vi "MB Param redefine.vi"(6 "conninfo":T1={"host"="localhost", "port"="5432", "client_encoding"="WIN1251", "dbname"="data", "user"="postgres", "password"=""}, 8 "error in (no error)":errorcluster, 9 "KFMTable":string="kfm_3", 10 "KFM param":string[](array[string]), 11 "MBs":refnum<class "Modbus Master CR.lvclass">[](array[class])) -> (0 "error":errorcluster, 3 "MBs out":refnum<class "Modbus Master CR.lvclass">[](array[class]))   [LabVIEW 2021]
uses:
  PostgreSQL/PostgreSQL2LabVIEW/ctl/Coninfo.ctl
  MB/Modbus Master CR.lvclass
  MBTCP Param/Typedefs/KFMParamColumns.ctl
  MBTCP Param/MBTCP Param.lvclass
  D:/my_projects/projects/Algorithms/Labview/21/Modbus_v2/MB Param/MB Param/MB Param.lvclass
  MB/Modbus Master CR.lvclass/Modbus Master CR.ctl
  MB Param.lvclass/MB Param.ctl
  MBTCP Param/MBTCP Param.lvclass/MBTCP Param.ctl
  MB Param.lvclass
  PostgreSQL/PostgreSQL2LabVIEW/libpqUtility/libpqutility.lvlib
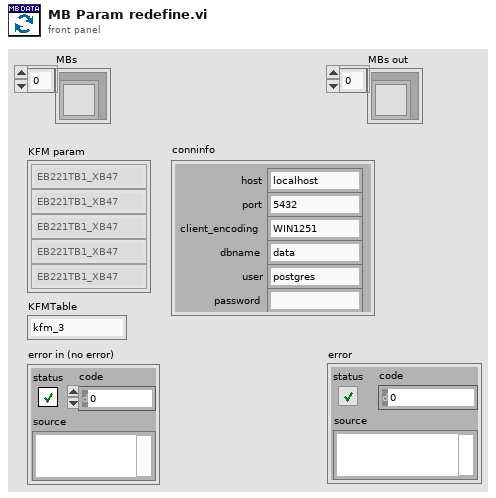
[diagram p1: front panel]
types:
  T1 = typedef "libpqutility.lvlib/Coninfo.ctl" = cluster{"host":string, "port":string, "client_encoding":string, "dbname":string, "user":string, "password":string}
  T2 = typedef "MBParam.lvlib/MBTCP Param.lvclass/KFMParamColumns.ctl" = enum16{"MVIName", "ip_adress", "port", "connection_timeout", "reconnection_timeout", "n_attempt_max", "reset_connect_timeout", "write_timeout", "read_timeout", "period", "enable", "write_enable", "fcode_full"}
  T3 = typedef "MBParam.lvlib/MBTCP Param.lvclass/timeouts.ctl" = cluster{"conn_timeout":i32, "reconn_timeout":i32, "N attempt max":i32, "t_reset_TTL":i32, "write_timeout":i32, "read_timeout":i32, "period":i32}
  T4 = cluster{"Remote IP Address":string, "Remote Port":u16}[]
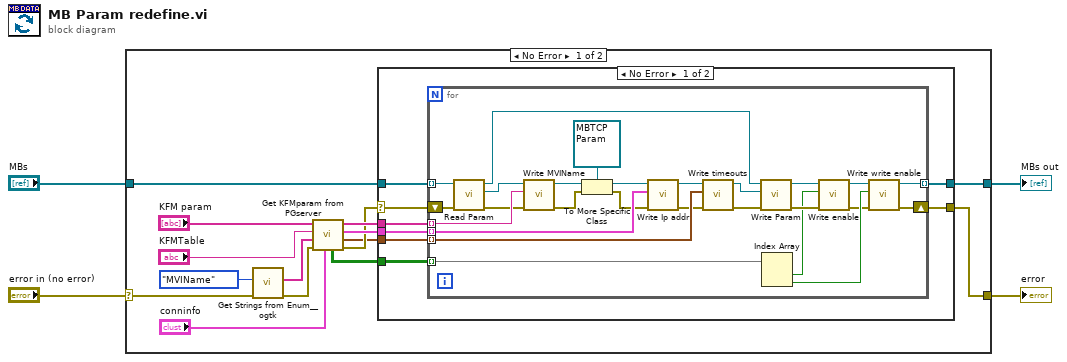
[diagram p0: block diagram]
diagram:
  n1 = case shown="No Error" "error in (no error)" {
    selector: "error in (no error)" -> [w9 w57]
    tunnel: [w19 w57] -> w4
    tunnel: "MBs" -> [w7 w56]
    tunnel: [w6 w56] -> w1
    frame No Error {
      n2 = call <userlib>:"Get Strings from Enum__ogtk.vi"("error in (no error)"=w9, "Enum"=KFMParamColumns."MVIName" ("KFMParamColumns")) -> ("error out"=w8:errorcluster, "Enum Strings"=w10:string[])  [unwired: 6 in, 2 out]
      n3 = call "Get KFMparam from PGserver.vi"("conninfo"="conninfo", "error in (no error)"=w8, "KFMParamColumns"=w10, "KFMParamTable"="KFMTable", "KFMParameters"="KFM param") -> ("error out"=w15:errorcluster, "timeouts"=w12:T3[], "IP Address"=w16:T4, "MVIName"=w17:string[], "enable"=w11:bool[][])  [unwired: 2 in]
      n4 = case shown="No Error" w15 {
        selector: w15 -> [w26 w55]
        tunnel: w17 -> [w23 _]
        tunnel: w16 -> [w25 _]
        tunnel: [w20 w55] -> w19
        tunnel: w12 -> [w24 _]
        tunnel: w11 -> [w22 _]
        tunnel: w7 -> [w27 w54]
        tunnel: [w21 w54] -> w6
        frame No Error {
          n5 = for {
            tunnel: w27 -> [w53] mode=indexing
            tunnel: w25 -> [w34] mode=indexing
            tunnel: w24 -> [w31] mode=indexing
            tunnel: w23 -> [w49] mode=indexing
            tunnel: w22 -> [w43] mode=indexing
            tunnel: [w39] -> w21 mode=indexing
            shift-right: [w38] -> w20
            shift-left: w26 -> [w52]
            n6 = call "Read Param.vi"("error in (no error)"=w52, "MB_TCP in"=w53) -> ("error out"=w47:errorcluster, "Param"=w50:refnum<class "MB Param.lvclass">, "MB_TCP out"=w46:refnum<class "Modbus Master CR.lvclass">)  [unwired: 7 in]
            n7 = call "Write MVIName.vi"("error in (no error)"=w47, "MVIName"=w49, "MB Param in"=w50) -> ("error out"=w36:errorcluster, "MB Param out"=w48:refnum<class "MB Param.lvclass">)  [unwired: 7 in]
            n8 = To More Specific Class(target class=refnum<class "MBTCP Param.lvclass"> refnum ("MBParam.lvlib:MBTCP Param.lvclass"), reference=w48, error in=w36) -> (specific class reference=w35:refnum<class "MBTCP Param.lvclass">, error out=w33:errorcluster)
            n9 = call "Write Ip addr.vi"("error in (no error)"=w33, "IP address"=w34, "MB Param in"=w35) -> ("error out"=w30:errorcluster, "MB Param out"=w32:refnum<class "MBTCP Param.lvclass">)  [unwired: 7 in]
            n10 = call "Write timeouts.vi"("error in (no error)"=w30, "timeouts"=w31, "MB Param in"=w32) -> ("error out"=w29:errorcluster, "MB Param out"=w28:refnum<class "MBTCP Param.lvclass">)  [unwired: 7 in]
            n11 = call "Write Param.vi"("error in (no error)"=w29, "Param"=w28, "MB_TCP in"=w46) -> ("error out"=w44:errorcluster, "MB_TCP out"=w45:refnum<class "Modbus Master CR.lvclass">)  [unwired: 7 in]
            n12 = Index Array(array=w43) -> (element #1=w42:bool, element #2=w41:bool)  [unwired: 2 in]
            n13 = call "Write enable.vi"("error in (no error)"=w44, "enable"=w42, "MB in"=w45) -> ("error out"=w40:errorcluster, "MB out"=w51:refnum<class "Modbus Master CR.lvclass">)  [unwired: 7 in]
            n14 = call "Write write enable.vi"("error in (no error)"=w40, "write enable"=w41, "MB in"=w51) -> ("error out"=w38:errorcluster, "MB out"=w39:refnum<class "Modbus Master CR.lvclass">)  [unwired: 7 in]
          }
        }
        frame Error {
        }
      }
    }
    frame Error {
    }
  }
  "error" <- w4
  "MBs out" <- w1
